vi "Core Read DAQ FIFO.vi"(7 "Release Lock":bool=TRUE, 8 "error in (no error)":errorcluster, 9 "Timeout (ms)":i32=100, 10 "DAQ In":T1[](array[typedef]), 11 "CIFTag in":refnum<class "CIF_NIChn_Fifo_DAQ.lvclass">) -> (0 "error out":errorcluster, 1 "timed out?":bool, 2 "DAQ Out":T1[](array[typedef]), 3 "CIFTag out":refnum<class "CIF_NIChn_Fifo_DAQ.lvclass">, 4 "Header":T2)   [LabVIEW 2021, in "CIF_NIChn_Fifo_DAQ.lvclass"]
uses:
  CIF_NIChn_Fifo_DAQ.lvclass
  D:/dev/Packages/Channel_Manager/src/CIFChannels/CIFChannels.lvclass
  D:/dev/Packages/Channel_Manager/src/CIF_NIChn/NIChn/CIF_NIChn.lvclass
  ChannelCommon/typedef/FIFO Header.ctl
  ChannelCommon/typedef/Datatype Waveform.ctl
  CIFChannels/CIFChannels.lvclass/CIFChannels.ctl
  NIChn/CIF_NIChn.lvclass/CIF_NIChn.ctl
  CIF_NIChn_Fifo_DAQ.lvclass/CIF_NIChn_Fifo_DAQ.ctl
  <vilib>/CIF Foundation/CIF Utilities/Statistics/I64/Stats_I64_CIF_U.lvclass/Stats_I64_CIF_U.ctl
  a66d495f-c29f-4596-8ad9-13e7f334244d.vi
  010c5156-5ad7-4e56-b6b0-a69033aca011.vi
  <vilib>/CIF Foundation/CIF Utilities/Time/System Time/Get System Time.vi
  <vilib>/CIF Foundation/CIF Utilities/Statistics/I64/X1 minus X0.vi
  NIChn/Accessors/Read CIF Channel.vi
  NIChn/SubVIs/Check Disconnect.vi
  <vilib>/CIFChannels/Top Level/Read Variable Length U8 Array.vi
  NIChn/Accessors/Write CIF Channel.vi
  Unflatten.vi
  CIFChannels/Utilities/Update Channel Benchmark.vi
  Core Read DAQ DVR FIFO.vi/e6dc5e5d-6043-485e-a6bf-7c23d051166d.vi
  Core Read DAQ DVR FIFO.vi/66a3f3ff-bc1e-4ae7-83d8-3035fbf2cfec.vi
  CIFChannels/Accessors/Read Channel State.vi
  CIFChannels/Accessors/Read Direction.vi
  <vilib>/CIF Foundation/CIF Utilities/Time/System Time/LabVIEW Time to TAI Time.vi
  <vilib>/CIF Foundation/CIF Utilities/Statistics/I64/X1 minus X0.vi/dfabcf33-0dbc-4041-80a5-3dc0c86d2989.vi
  CIFChannels/Accessors/Write Channel State.vi
  CIFChannels/Accessors/Read Tag Disconnect Behavior.vi
  <vilib>/CIFChannels/Top Level/Read Variable Length U8 Array.vi/81056090-23cf-424a-a716-29db01c8ef1b.vi
  <vilib>/CIFChannels/Top Level/Read Variable Length U8 Array.vi/6610cd62-0a6d-4591-8fd4-6453482a4bc1.vi
  <vilib>/CIFChannels/Top Level/Read Variable Length U8 Array.vi/93d598b0-524b-4f76-9570-a74a86ef2c6f.vi
  ChannelCommon/CIFFIFO/Flatten/DVR Unflatten.vi
  CIFChannels/Accessors/Write FIFO Header.vi
  CIFChannels/Accessors/Write FIFO Timeout.vi
  <vilib>/CIF Foundation/CIF Utilities/Statistics/I64/X1 minus X0.vi/dfabcf33-0dbc-4041-80a5-3dc0c86d2989.vi/9eb60a9a-770f-4d2d-8b3f-8465c267ecc9.vi
  <vilib>/CIFChannels/Top Level/Read Variable Length U8 Array.vi/81056090-23cf-424a-a716-29db01c8ef1b.vi/4bc1c15b-36ab-481f-b8dd-c64075ce723a.vi
  <vilib>/CIFChannels/Top Level/Read Variable Length U8 Array.vi/81056090-23cf-424a-a716-29db01c8ef1b.vi/d83cb72b-7713-41fc-a3d1-682de79cf574.vi
  <vilib>/CIFChannels/SubVIs/Get dll Path.vi
  <vilib>/CIFChannels/Top Level/Read Variable Length U8 Array.vi/6610cd62-0a6d-4591-8fd4-6453482a4bc1.vi/c28b0ead-42ad-4072-80a2-aca7f2bd7ce3.vi
  <vilib>/CIFChannels/Top Level/Read Variable Length U8 Array.vi/93d598b0-524b-4f76-9570-a74a86ef2c6f.vi/4bc1c15b-36ab-481f-b8dd-c64075ce723a.vi
  <vilib>/CIFChannels/Top Level/Read Variable Length U8 Array.vi/93d598b0-524b-4f76-9570-a74a86ef2c6f.vi/d83cb72b-7713-41fc-a3d1-682de79cf574.vi
  ChannelCommon/Utilities/Unflatten Header.vi
  ChannelCommon/Utilities/Add Error.vi
  <vilib>/CIF Foundation/CIF Utilities/DataTypes/Unflatten U64.vi
  <vilib>/CIF Foundation/CIF Utilities/DataTypes/Unflatten I64.vi
  <vilib>/CIF Foundation/CIF Utilities/Errors/Append Error Location.vi
  NIChn/CIF_NIChn.lvclass
  ChannelCommon/ChannelCommon.lvlib
  CIFChannels/CIFChannels.lvclass
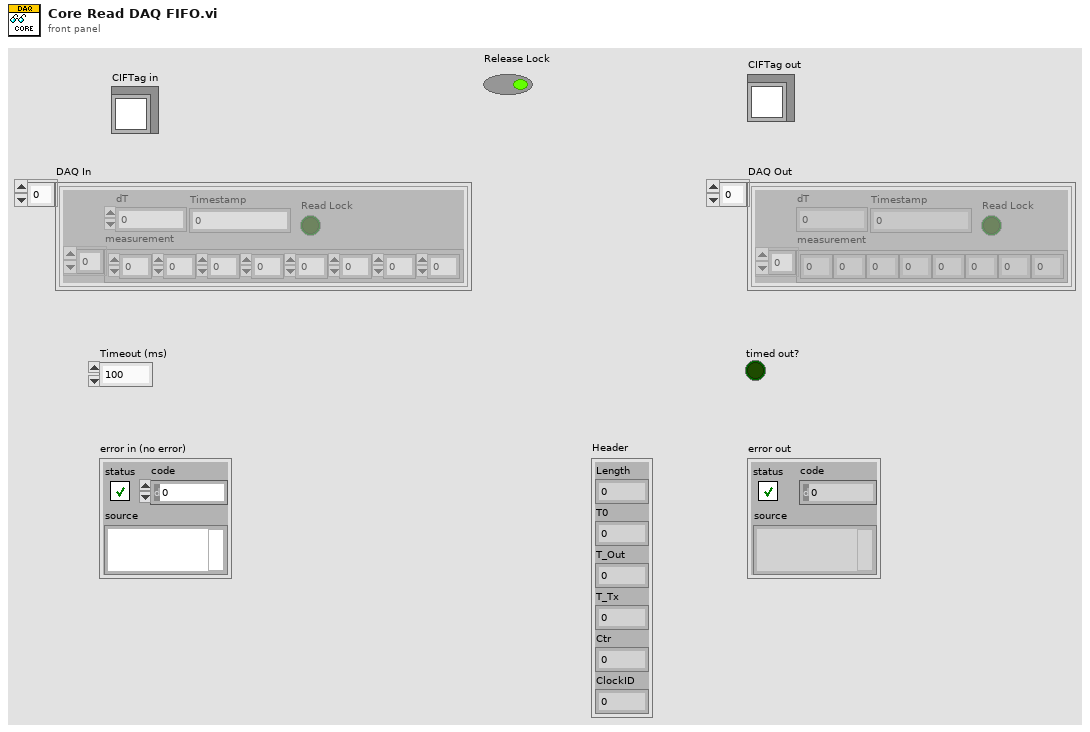
[diagram p1: front panel]
types:
  T1 = typedef "ChannelCommon.lvlib/Datatype Waveform.ctl" = cluster{"measurement":dbl[], "dT":dbl, "Timestamp":i64, "Read Lock":bool}
  T2 = typedef "ChannelCommon.lvlib/FIFO Header.ctl" = cluster{"Length":u64, "T0":i64, "T_Out":i64, "T_Tx":i64, "Ctr":u64, "ClockID":u8}
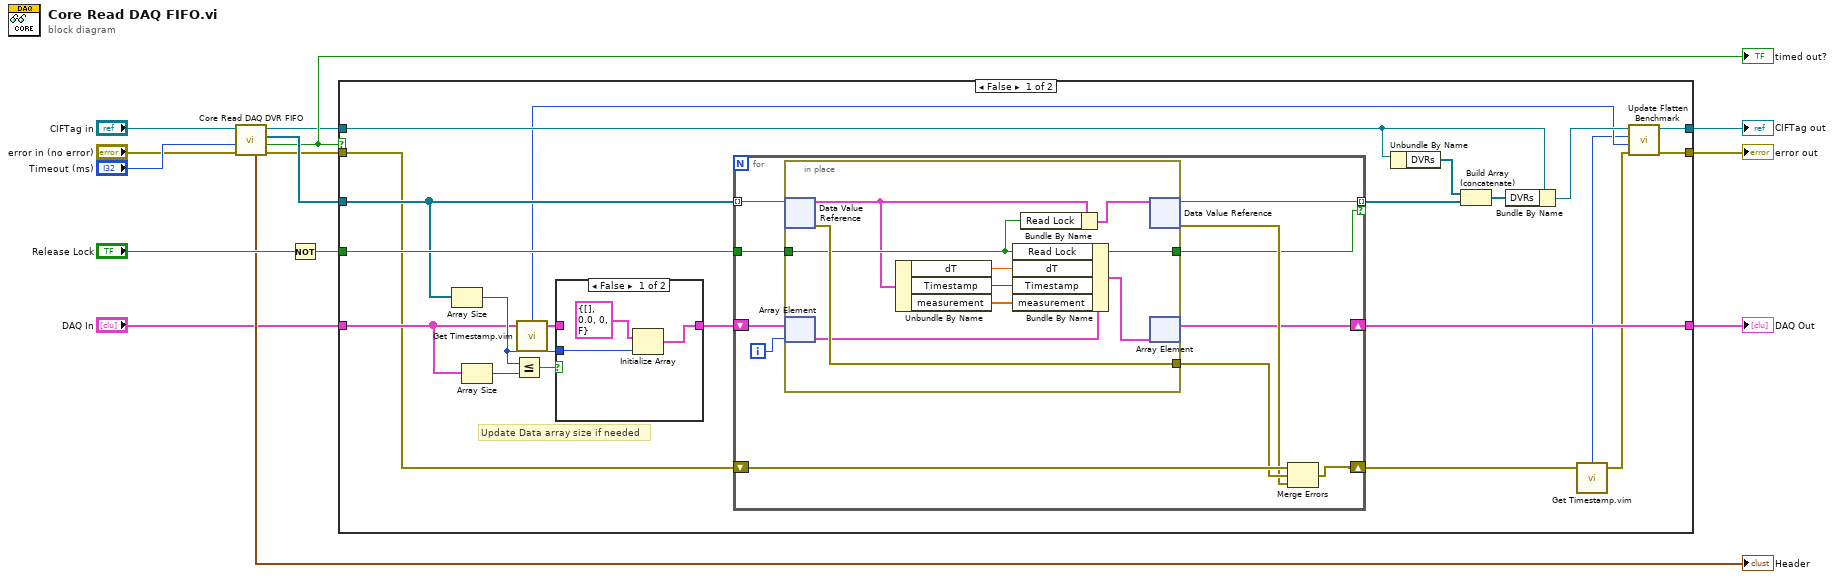
[diagram p0: block diagram]
diagram:
  n1 = call "Core Read DAQ DVR FIFO.vi"("error in (no error)"="error in (no error)", "Timeout (ms)"="Timeout (ms)", "CIFTag in"="CIFTag in") -> ("error out"=w3:errorcluster, "timed out?"=w11:bool, "Data Out"=w14:refnum<data-value>[], "CIFTag out"=w4:refnum<class "CIF_NIChn_Fifo_DAQ.lvclass">, "Header"=→"Header":T2)  [unwired: 4 in]
  "timed out?" <- w11
  n2 = Not(x="Release Lock") -> (.not. x?=w12:bool)
  n3 = case shown="False" w11 {
    tunnel: w3 -> [w16 w62]
    tunnel: w14 -> [w30 _]
    tunnel: [w20 w62] -> w1
    tunnel: "DAQ In" -> [w18 w61]
    tunnel: w12 -> [w35 _]
    tunnel: [w34 w61] -> w7
    tunnel: w4 -> [w24 w60]
    tunnel: [w22 w60] -> w2
    frame False {
      # "Update Data array size if needed"
      n4 = Array Size(array=w30) -> (size(s)=w29:i32)
      n5 = Array Size(array=w18) -> (size(s)=w32:i32)
      n6 = Less Or Equal?(x=w29, y=w32) -> (x <= y?=w33:bool)
      n7 = call "Get Timestamp.vim"("Anything in"=w18) -> ("Time (ns)"=w19:i64, "Anything out"=w17:T1[])  [unwired: 2 in]
      n8 = case shown="False" w33 {
        tunnel: w17 -> [_ w39]
        tunnel: [w36 w39] -> w31
        tunnel: w29 -> [w38 _]
        frame False {
          n9 = Initialize Array(T1 {"measurement"=[], "dT"=0.0, "Timestamp"=0, "Read Lock"=FALSE} ("Waveform Datatype"), w38) -> (w36:T1[])
        }
        frame True {
        }
      }
      n10 = for {
        tunnel: w30 -> [w50] mode=indexing
        shift-right: [w46] -> w28
        shift-left: w16 -> [w49]
        shift-right: [w41] -> w34
        shift-left: w31 -> [w42]
        tunnel: w35 -> [w45]
        tunnel: [w44] -> w25 mode=indexing if=w43
        i -> [w40]
        n11 = in-place {
          in-place-border: [w59] -> w48
          in-place-border: w45 -> [w57]
          in-place-border: [w57] -> w43
          n12 = in-place-dvr #1(w50) -> (w51:T1, w59:errorcluster)
          n13 = in-place-array #2(w42, w40) -> (w53:T1)
          n14 = Unbundle By Name(w51) -> ("dT"=w54:dbl, "Timestamp"=w55:i64, "measurement"=w56:dbl[])
          n15 = Bundle By Name(cluster=w53, "Read Lock"=w57, "dT"=w54, "Timestamp"=w55, "measurement"=w56) -> (w52:T1)
          n16 = Bundle By Name(cluster=w51, "Read Lock"=w57) -> (w58:T1)
          n17 = in-place-dvr #1(w58) -> (w44:refnum<data-value>, w47:errorcluster)
          n18 = in-place-array #2(w52) -> (w41:T1[])  [unwired: 1 out]
        }
        n19 = Merge Errors(w49, w48, w47) -> (w46:errorcluster)
      }
      n20 = Unbundle By Name(w24) -> ("DVRs"=w26:refnum<data-value>[])
      n21 = Build Array (concatenate)(w26, w25) -> (w27:refnum<data-value>[])
      n22 = Bundle By Name(cluster=w24, "DVRs"=w27) -> (w23:refnum<class "CIF_NIChn_Fifo_DAQ.lvclass">)
      n23 = call "Get Timestamp.vim"("Anything in"=w28) -> ("Time (ns)"=w15:i64, "Anything out"=w21:errorcluster)  [unwired: 2 in]
      n24 = call "Update Flatten Benchmark.vi"("error in (no error)"=w21, "X0"=w19, "X1"=w15, "CIFChannels in"=w23) -> ("error out"=w20:errorcluster, "CIFChannels out"=w22:refnum<class "CIF_NIChn_Fifo_DAQ.lvclass">)  [unwired: 6 in]
    }
    frame True {
    }
  }
  "error out" <- w1
  "CIFTag out" <- w2
  "DAQ Out" <- w7
